vi "Center Callee in Window Bounds.vi"(8 "Error In":errorcluster, 10 "Callee VI Refnum (Caller)":refnum<vi>, 11 "Block Diagram Window:Window Bounds":T1) -> (0 "Error Out":errorcluster)   [LabVIEW 2017, in "csm-tool-support.lvlib"]
doc: "This VI is designed to center a callee VI's window in a caller VI's window.\n\nAuthored by Brandon Steele\nsupport@mooregoodideas.com\nwww.mooregoodideas.com\n\nCopyright (c) 2010, Moore Good Ideas, Inc.\n\nAll rights reserved.\n\nRedistribution and use in source and binary forms, with or without modification, are permitted provided that the following conditions are met:\n\n * Redistributions of source code must retain the above copyright notice, this list of conditions and the following disclaimer.\n * Redistributions in binary form must reproduce the above copyright notice, this list of conditions and the following disclaimer in the documentation and/or other materials provided with the distribution.\n * Neither the name of Moore Good Ideas, Inc. nor the names of its contributors may be used to endorse or promote products derived from this software without specific prior written permission.\n\nTHIS SOFTWARE IS PROVIDED BY THE COPYRIGHT HOLDERS AND CONTRIBUTORS \"AS IS\" AND ANY EXPRESS OR IMPLIED WARRANTIES, INCLUDING, BUT NOT LIMITED TO, THE IMPLIED WARRANTIES OF MERCHANTABILITY AND FITNESS FOR A PARTICULAR PURPOSE ARE DISCLAIMED. IN NO EVENT SHALL THE COPYRIGHT OWNER OR CONTRIBUTORS BE LIABLE FOR ANY DIRECT, INDIRECT, INCIDENTAL, SPECIAL, EXEMPLARY, OR CONSEQUENTIAL DAMAGES (INCLUDING, BUT NOT LIMITED TO, PROCUREMENT OF SUBSTITUTE GOODS OR SERVICES; LOSS OF USE, DATA, OR PROFITS; OR BUSINESS INTERRUPTION) HOWEVER CAUSED AND ON ANY THEORY OF LIABILITY, WHETHER IN CONTRACT, STRICT LIABILITY, OR TORT (INCLUDING NEGLIGENCE OR OTHERWISE) ARISING IN ANY WAY OUT OF THE USE OF THIS SOFTWARE, EVEN IF ADVISED OF THE POSSIBILITY OF SUCH DAMAGE."
uses:
  csm-tool-support.lvlib
  <vilib>/Utility/miscctls.llb/LVRectTypeDef.ctl
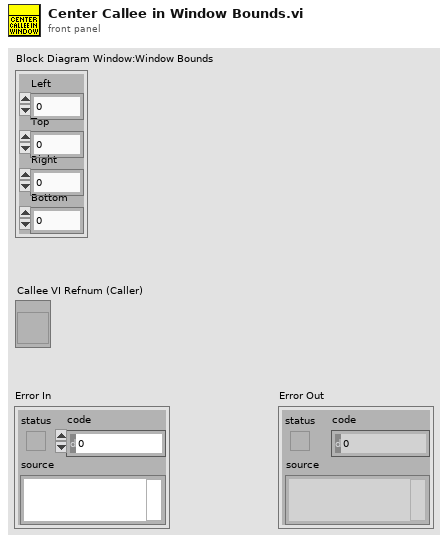
[diagram p1: front panel]
types:
  T1 = typedef "LVRectTypeDef.ctl" = cluster{"Left":i16, "Top":i16, "Right":i16, "Bottom":i16}
  T2 = cluster{"Left":bool, "Top":bool, "Right":bool, "Bottom":bool}
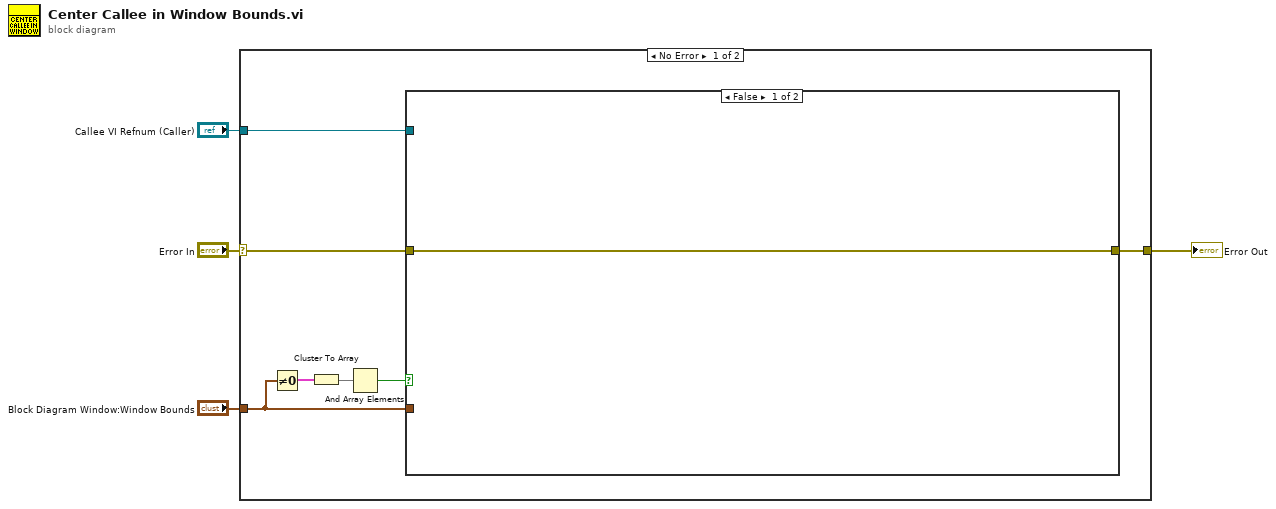
[diagram p0: block diagram]
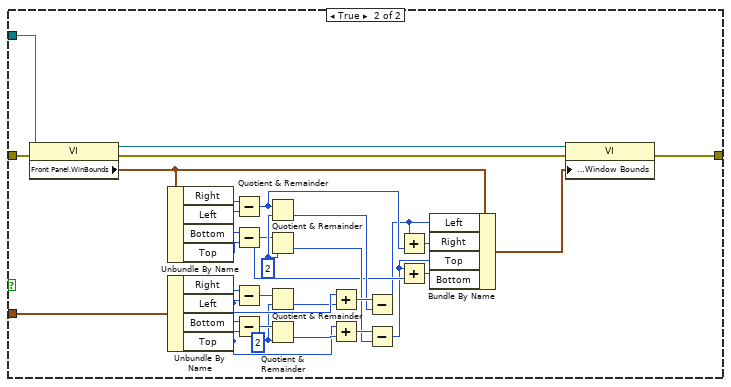
[diagram p2: hidden frame]
diagram:
  n1 = case shown="No Error" "Error In" {
    selector: "Error In" -> [w10 w45]
    tunnel: [w11 w45] -> w4
    tunnel: "Block Diagram Window:Window Bounds" -> [w8 _]
    tunnel: "Callee VI Refnum (Caller)" -> [w9 _]
    frame No Error {
      n2 = Not Equal To 0?(x=w8) -> (x != 0?=w7:T2)
      n3 = Cluster To Array(cluster=w7) -> (array=w6:bool[])
      n4 = And Array Elements(Boolean array=w6) -> (logical AND=w5:bool)
      n5 = case shown="False" w5 {
        tunnel: [w12 w44] -> w11
        tunnel: w10 -> [w12 w21]
        tunnel: w9 -> [_ w20]
        tunnel: w8 -> [_ w13]
        frame False {
        }
        frame True {
          w39 = i16 2 ("y")
          w22 = i16 2 ("y")
          n6 = property class="VI"(reference=w20, error in=w21) -> (reference out=w26:refnum<vi>, error out=w25:errorcluster, "Front Panel.WinBounds"=w15:T1)
          n7 = Unbundle By Name(w15) -> ("Right"=w35:i16, "Left"=w36:i16, "Bottom"=w37:i16, "Top"=w38:i16)
          n8 = Unbundle By Name(w13) -> ("Right"=w43:i16, "Left"=w34:i16, "Bottom"=w42:i16, "Top"=w31:i16)
          n9 = Subtract(x=w35, y=w36) -> (x-y=w24:i16)
          n10 = Subtract(x=w37, y=w38) -> (x-y=w23:i16)
          n11 = Subtract(x=w43, y=w34) -> (x-y=w41:i16)
          n12 = Subtract(x=w42, y=w31) -> (x-y=w40:i16)
          n13 = Quotient & Remainder(x=w24, y=w39) -> (floor(x/y)=w29:i16)  [unwired: 1 out]
          n14 = Quotient & Remainder(x=w23, y=w39) -> (floor(x/y)=w27:i16)  [unwired: 1 out]
          n15 = Quotient & Remainder(x=w41, y=w22) -> (floor(x/y)=w33:i16)  [unwired: 1 out]
          n16 = Quotient & Remainder(x=w40, y=w22) -> (floor(x/y)=w32:i16)  [unwired: 1 out]
          n17 = Add(x=w34, y=w33) -> (x+y=w30:i16)
          n18 = Add(x=w31, y=w32) -> (x+y=w28:i16)
          n19 = Subtract(x=w30, y=w29) -> (x-y=w18:i16)
          n20 = Subtract(x=w28, y=w27) -> (x-y=w17:i16)
          n21 = Add(x=w18, y=w24) -> (x+y=w16:i16)
          n22 = Add(x=w17, y=w23) -> (x+y=w19:i16)
          n23 = Bundle By Name(cluster=w15, "Left"=w18, "Right"=w16, "Top"=w17, "Bottom"=w19) -> (w14:T1)
          n24 = property class="VI"(reference=w26, error in=w25, "Front Panel Window:Window Bounds"=w14) -> (error out=w44:errorcluster)  [unwired: 1 out]
        }
      }
    }
    frame Error {
    }
  }
  "Error Out" <- w4
